vi "sin_point.vi"(9 "Time":dbl format="%#_13g", 10 "Amplitude":dbl format="%#_13g", 11 "Frequency":dbl format="%#_13g") -> (3 "Output":dbl)   [LabVIEW 2016]
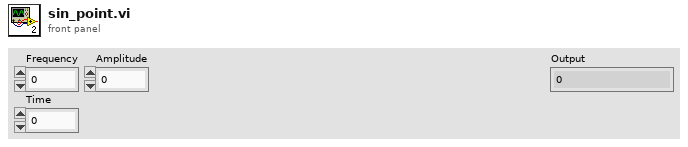
[diagram p1: front panel]
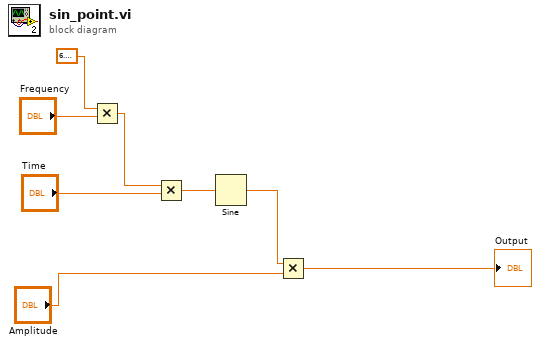
[diagram p0: block diagram]
diagram:
  n1 = Multiply(x=6.283185307179586, y="Frequency") -> (x*y=w5:dbl)
  n2 = Multiply(x=w5, y="Time") -> (x*y=w4:dbl)
  n3 = Sine(x=w4) -> (sin(x)=w3:dbl)
  n4 = Multiply(x=w3, y="Amplitude") -> (x*y=→"Output":dbl)
